vi "Measure.vi"(0 "Serial port":refnum<visa-resource-name>, 1 "Device":u8=1) -> (3 "Serial port out":refnum<visa-resource-name>, 4 "Device out":u8=1, 5 "Voltage":sgl, 6 "Current":sgl)   [LabVIEW 2021]
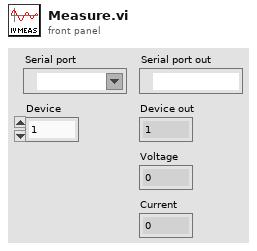
[diagram p1: front panel]
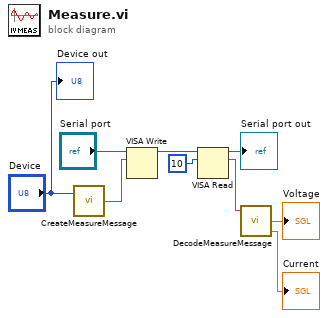
[diagram p0: block diagram]
diagram:
  n1 = call "CreateMeasureMessage.vi"("Device"="Device") -> ("Message"=w5:string)  [unwired: 1 in]
  n2 = VISA Write(VISA resource name="Serial port", write buffer=w5) -> (VISA resource name out=w9:refnum<visa-resource-name>)  [unwired: 1 in, 2 out]
  n3 = VISA Read(VISA resource name=w9, byte count=u32 10) -> (VISA resource name out=→"Serial port out":refnum<visa-resource-name>, read buffer=w4:string)  [unwired: 1 in, 2 out]
  n4 = call "DecodeMeasureMessage.vi"("Message"=w4) -> ("Current"=→"Current":sgl, "Voltage"=→"Voltage":sgl)  [unwired: 2 in, 1 out]
  "Device out" <- "Device"
